vi "niDTS WLAN INSTR TX Configure SEM.vi"(8 "error in (no error)":errorcluster, 11 "niDTS WLAN INSTR TX in":refnum<class "niDTS WLAN INSTR TX.lvclass">) -> (0 "error out":errorcluster, 3 "niDTS WLAN INSTR TX out":refnum<class "niDTS WLAN INSTR TX.lvclass">)   [LabVIEW 2015, in "niDTS WLAN.lvlib" / "niDTS WLAN INSTR TX.lvclass"]
doc: "Sets:\n\n* SpectralMaskEnabled\n* NumberOfAverages(sem)\n* AutoSpanEnabled\n* FrequnecySpan"
uses:
  niDTS WLAN INSTR TX.lvclass
  niDTS WLAN INSTR TX.lvclass/niDTS WLAN INSTR TX.ctl
  RiviInstDriver/niRfsaWlan/Objects/niRfsaWlan.lvclass
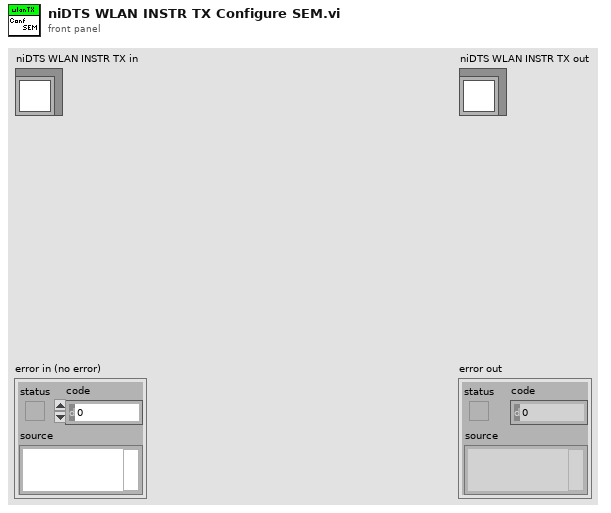
[diagram p1: front panel]
types:
  T1 = typedef "niRfsaWlan.lvclass/niRfsaWlan INC Handle.ctl" = refnum<data-value>
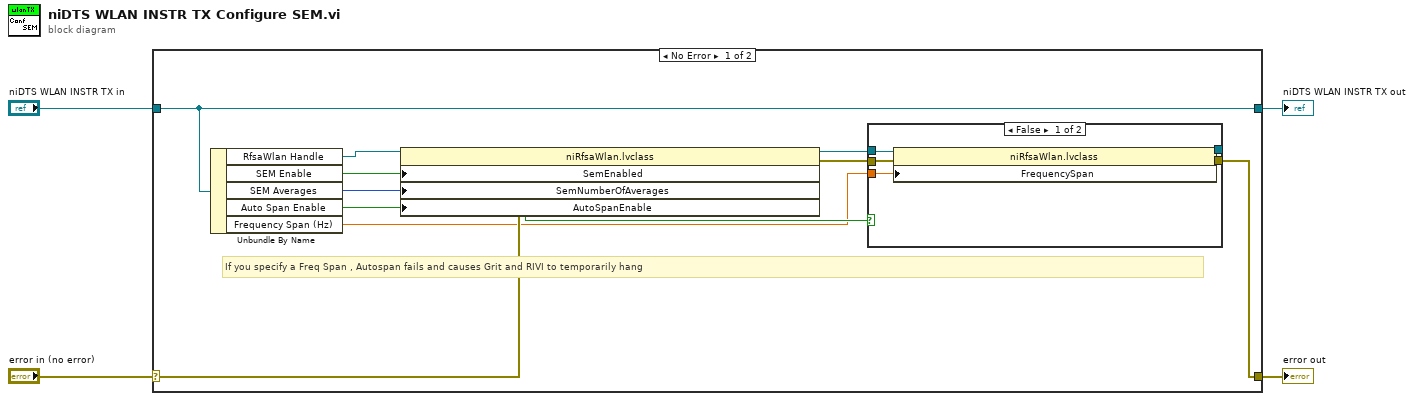
[diagram p0: block diagram]
diagram:
  n1 = case shown="No Error" "error in (no error)" {
    selector: "error in (no error)" -> [w11 w23]
    tunnel: [w5 w23] -> w3
    tunnel: [w14 w22] -> w1
    tunnel: "niDTS WLAN INSTR TX in" -> [w14 w22]
    frame No Error {
      # "If you specify a Freq Span , Autospan fails and causes Grit and RIVI to temporarily hang"
      n2 = Unbundle By Name(w14) -> ("RfsaWlan Handle"=w12:T1, "SEM Enable"=w9:bool, "SEM Averages"=w8:i32, "Auto Span Enable"=w7:bool, "Frequency Span (Hz)"=w6:dbl)
      n3 = property class="niRfsaWlan.lvclass"(reference=w12, error in=w11, "SemEnabled"=w9, "SemNumberOfAverages"=w8, "AutoSpanEnable"=w7) -> (reference out=w13:T1, error out=w10:errorcluster)
      n4 = case shown="False" w7 {
        tunnel: w6 -> [w19 _]
        tunnel: w13 -> [w18 w21]
        tunnel: w10 -> [w17 w20]
        tunnel: [w16 w21] -> _
        tunnel: [w15 w20] -> w5
        frame False {
          n5 = property class="niRfsaWlan.lvclass"(reference=w18, error in=w17, "FrequencySpan"=w19) -> (reference out=w16:T1, error out=w15:errorcluster)
        }
        frame True {
        }
      }
    }
    frame Error {
    }
  }
  "error out" <- w3
  "niDTS WLAN INSTR TX out" <- w1
